vi "RunOneTest.vi"(6 "ShowPanel? (f)":bool=TRUE, 7 ".tst file":path, 8 "Error Array In":errorcluster[](array[cluster]), 11 "TestTreeTags":string[](array[string])=["0_3_0_0_0_12_73_110_105_116_32_97_110_100_32_82_117_110_80_84_72_48_0_0_0_84_0_0_0_10_1_67_5_85_115_101_114_115_6_80_117_98_108_105_99_8_80_114_111_106_101_99_116_115_5_73_67_68_65_83_9_85_115_101_114_70_105_108_101_115_7_80_108_117_103_105_110_115_6_83_101_110_115_111_114_9_82_111_111_109_65_108_101_114_116_14_82_111_111_109_65_108_101_114_116_49_46_105_110_105_0_0_0_3_0_0_0_18_69_114_114_111_114_83_101_118_101_114_105_116_121_44_83_116_111_112_0_0_0_22_83_101_110_115_111_114_67_114_101_97_116_101_83_101_115_115_105_111_110_44_35_36_0_0_0_14_83_101_110_115_111_114_83_116_97_114_116_44_35_36", "0_3_0_0_0_12_73_110_105_116_32_97_110_100_32_82_117_110_80_84_72_48_0_0_0_98_0_0_0_10_1_67_5_85_115_101_114_115_6_80_117_98_108_105_99_8_80_114_111_106_101_99_116_115_5_73_67_68_65_83_9_85_115_101_114_70_105_108_101_115_7_80_108_117_103_105_110_115_6_83_101_110_115_111_114_28_83_105_101_109_101_110_115_32_68_105_103_105_116_97_108_32_69_110_101_114_103_121_32_77_101_116_101_114_9_83_68_69_77_48_46_105_110_105_0_0_0_3_0_0_0_18_69_114_114_111_114_83_101_118_101_114_105_116_121_44_83_116_111_112_0_0_0_22_83_101_110_115_111_114_67_114_101_97_116_101_83_101_115_115_105_111_110_44_35_36_0_0_0_14_83_101_110_115_111_114_83_116_97_114_116_44_35_36"]) -> (0 "ErrorArray Out":errorcluster[](array[cluster]), 1 "TDMS Log File":path)   [LabVIEW 2018]
uses:
  NistPluggableModules/TestClass/Test.lvclass/Test.ctl
  NistPluggableModules/TestClass/Accessors/Read ModuleList.vi
  NistPluggableModules/TestClass/Test.lvclass
  <userlib>/NIST/NISTErrorLib/NISTErrorLib.lvlib
  NistPluggableModules/Visualization/VisualizeBase/VisualizeBase_class/VisualizeBase.lvclass
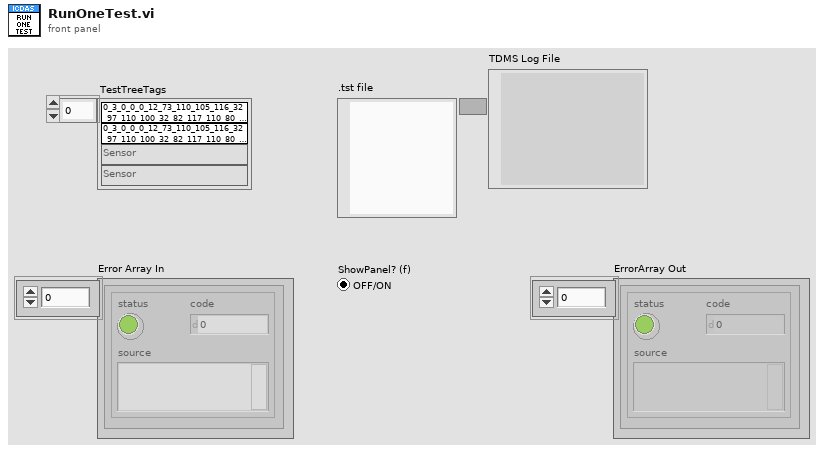
[diagram p1: front panel]
types:
  T1 = typedef "Plugin Tree Tag.ctl" = cluster{"ItemType":T2, "Name":string, "Path":path, "Script":string[]}
  T2 = typedef "Plugins Tree Item Type.ctl" = enum16{"Plugin", "Instrument", "INI File", "INI Script"}
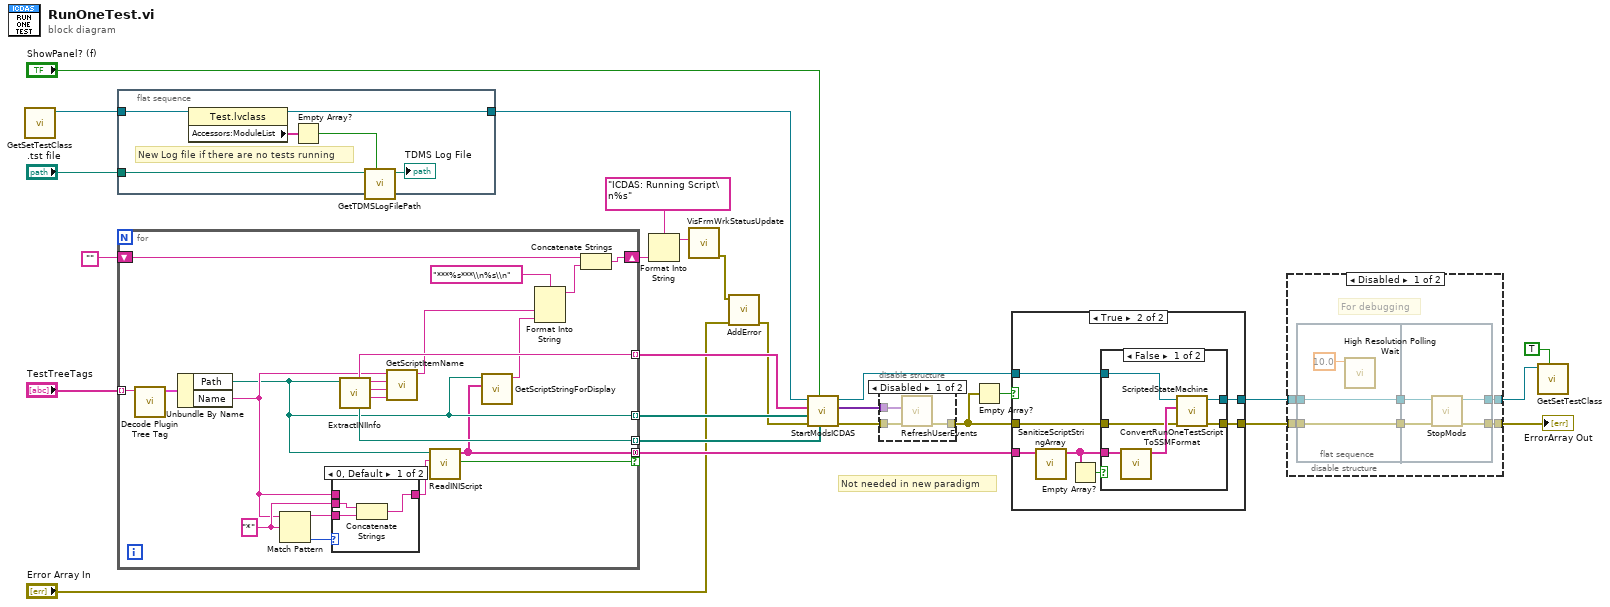
[diagram p0: block diagram]
diagram:
  # "Not needed in new paradigm"
  n1 = call "GetSetTestClass.vi"() -> ("Test.lvclass"=w14:refnum<class "Test.lvclass">)  [unwired: 11 in]
  n2 = flat-sequence {
    tunnel: w14 -> [w32]
    tunnel: [w31] -> w10
    tunnel: ".tst file" -> [w29]
    frame #0 {
      # "New Log file if there are no tests running"
      n3 = property class="Test.lvclass"(reference=w32) -> (reference out=w31:refnum<class "Test.lvclass">, "Accessors:ModuleList"=w30:string[])  [unwired: 1 in, 1 out]
      n4 = Empty Array?(array=w30) -> (empty?=w27:bool)
      n5 = call "GetTDMSLogFilePath.vi"("Set? (F)"=w27, ".tst file"=w29) -> ("TDMS Log File Path"=→"TDMS Log File":path)  [unwired: 9 in]
    }
  }
  n6 = for {
    tunnel: "TestTreeTags" -> [w53] mode=indexing
    tunnel: [w36] -> w12 mode=indexing
    tunnel: [w51] -> w11 mode=indexing
    tunnel: [w35] -> w20 mode=concatenating if=w45
    tunnel: [w50] -> w13 mode=indexing
    shift-right: [w37] -> w6
    shift-left: "" -> [w40]
    w47 = "*" ("regular expression")
    n7 = call "Decode Plugin Tree Tag.vi"("Tag"=w53) -> ("Plugin Tree Tag"=w52:T1)  [unwired: 9 in, 1 out]
    n8 = Unbundle By Name(w52) -> ("Path"=w36:path, "Name"=w41:string)
    n9 = Match Pattern(string=w41, regular expression=w47) -> (before substring=w48:string, offset past match=w49:i32)  [unwired: 1 in, 2 out]
    n10 = case shown="0, Default" w49 {
      tunnel: w41 -> [_ w57]
      tunnel: [w54 w57] -> w46
      tunnel: w48 -> [w56 _]
      tunnel: w47 -> [w55 _]
      frame 0, Default {
        n11 = Concatenate Strings(w55, w56) -> (w54:string)
      }
      frame 1 {
      }
    }
    n12 = call "ExtractINIInfo.vi"("INI File Path"=w36) -> ("INI File Name"=w42:string, "Class Name"=w43:string, "Module Name"=w44:string, "Visualization VI Path"=w50:path, "Module.Class.INI File Name"=w51:string)  [unwired: 4 in, 2 out]
    n13 = call "GetScriptItemName.vi"("INI File Name"=w42, "Class Name"=w43, "Module Name"=w44, "Script Name"=w41) -> ("Script Item Name"=w38:string)  [unwired: 6 in, 1 out]
    n14 = call "ReadINIScript.vi"("Script Name"=w46, "INI File Path"=w36) -> ("found?"=w45:bool, "Script"=w35:string[])  [unwired: 6 in, 2 out]
    n15 = call "GetScriptStringForDisplay.vi"("Script"=w35, "INI File Path"=w36) -> ("Script String"=w34:string)  [unwired: 9 in]
    n16 = Format Into String(format string="***%s***\\n%s\\n", w38, w34) -> (resulting string=w33:string)  [unwired: 2 in, 1 out]
    n17 = Concatenate Strings(w40, w33) -> (w37:string)
  }
  n18 = Format Into String(format string="ICDAS: Running Script\n%s", w6) -> (resulting string=w4:string)  [unwired: 2 in, 1 out]
  n19 = call "VisFrmWrkStatusUpdate.vi"("Status"=w4) -> ("error out"=w3:errorcluster)  [unwired: 10 in]
  n20 = call <userlib>:"AddError.vi"("ErrorArray In"="Error Array In", "error in (no error)"=w3) -> ("ErrorArray Out"=w1:errorcluster[])  [unwired: 8 in, 1 out]
  n21 = call "StartModsICDAS.vi"("Visualization VI Paths"=w13, "ShowPanel? (f)"="ShowPanel? (f)", "Error Array In"=w1, "INI File Paths"=w12, "Module List"=w11, "Test.lvclass"=w10) -> ("Error Array Out"=w16:errorcluster[], "Event Array"=w17:variant[], "Test.lvclass"=w25:refnum<class "Test.lvclass">)  [unwired: 3 in]
  n22 = disable-structure shown="Disabled" {
    disable-tunnel: w17 -> [w60 _]
    disable-tunnel: w16 -> [w59 w61]
    disable-tunnel: [w58 w61] -> w15
    frame Disabled {
      n23 = call "RefreshUserEvents.vi"("ErrorIn"=w59, "Data"=w60) -> ("ErrorOut"=w58:errorcluster[])  [unwired: 9 in]
    }
    frame Enabled {
    }
  }
  n24 = Empty Array?(array=w15) -> (empty?=w26:bool)
  n25 = case shown="True" w26 {
    tunnel: w25 -> [w63 w69]
    tunnel: [w63 w70] -> w24
    tunnel: w15 -> [w62 w68]
    tunnel: [w62 w67] -> w21
    tunnel: w20 -> [_ w66]
    frame False {
    }
    frame True {
      n26 = call "SanitizeScriptStringArray.vi"("Array in"=w66) -> ("Array out"=w65:string[])  [unwired: 10 in]
      n27 = Empty Array?(array=w65) -> (empty?=w64:bool)
      n28 = case shown="False" w64 {
        tunnel: [w75 w77] -> w70
        tunnel: w69 -> [w74 w77]
        tunnel: w68 -> [w73 w78]
        tunnel: [w72 w78] -> w67
        tunnel: w65 -> [w71 _]
        frame False {
          n29 = call "ConvertRunOneTestScriptToSSMFormat.vi"("Script in"=w71) -> ("Script out"=w76:string[])  [unwired: 10 in]
          n30 = call "ScriptedStateMachine.vi"("ErrorArray"=w73, "script"=w76, "Test.lvclass"=w74) -> ("ErrorArray"=w72:errorcluster[], "Test.lvclass"=w75:refnum<class "Test.lvclass">)  [unwired: 6 in, 1 out]
        }
        frame True {
          # "No script to run"
        }
      }
    }
  }
  n31 = disable-structure shown="Disabled" {
    disable-tunnel: w24 -> [w84 w93]
    disable-tunnel: w21 -> [w83 w92]
    disable-tunnel: [w82 w92] -> w23
    disable-tunnel: [w81 w93] -> w18
    frame Disabled {
      # "For debugging"
      n32 = flat-sequence {
        tunnel: w83 -> [w86]
        tunnel: w84 -> [w87]
        tunnel: [w87] -> w80
        tunnel: [w86] -> w79
        tunnel: [w89] -> w82
        tunnel: [w88] -> w81
        tunnel: w80 -> [w91]
        tunnel: w79 -> [w90]
        frame #0 {
          n33 = call <vilib>:"High Resolution Polling Wait.vi"("seconds to wait"=10.0) -> ()  [unwired: 10 in, 1 out]
        }
        frame #1 {
          n34 = call "StopMods.vi"("ErrorArray In"=w90, "Test.lvclass"=w91) -> ("ErrorArray Out"=w89:errorcluster[], "Test.lvclass"=w88:refnum<class "Test.lvclass">)  [unwired: 8 in]
        }
      }
    }
    frame Enabled {
    }
  }
  "ErrorArray Out" <- w23
  n35 = call "GetSetTestClass.vi"("Set"=TRUE, "Test.lvclass"=w18) -> ()  [unwired: 9 in, 1 out]
